vi "粗切.vi"() -> ()   [LabVIEW 2014]
panel:
  out "粗切项目":string
  out "粗切当前状态":string
  out "粗切条码":string
  out "粗切工位生产信息":string[][](table)
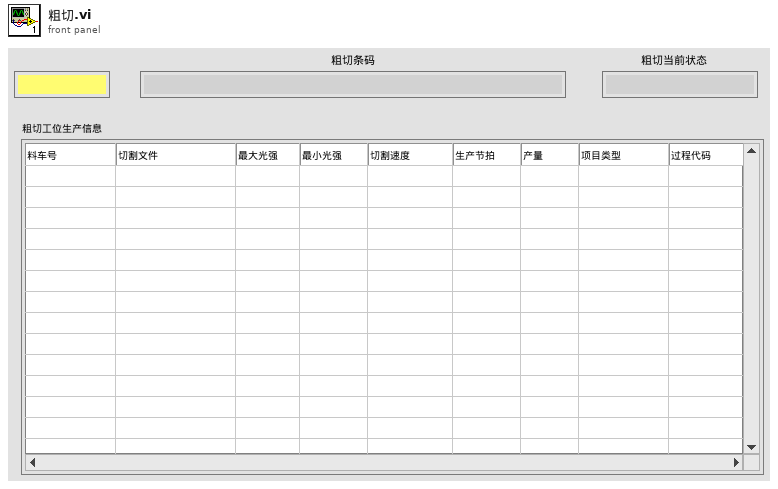
[diagram p1: front panel]
types:
  T1 = cluster{"粗切工位生产信息":refnum<vi>, "粗切条码":refnum<vi>, "粗切当前状态":refnum<vi>, "粗切项目":refnum<vi>}
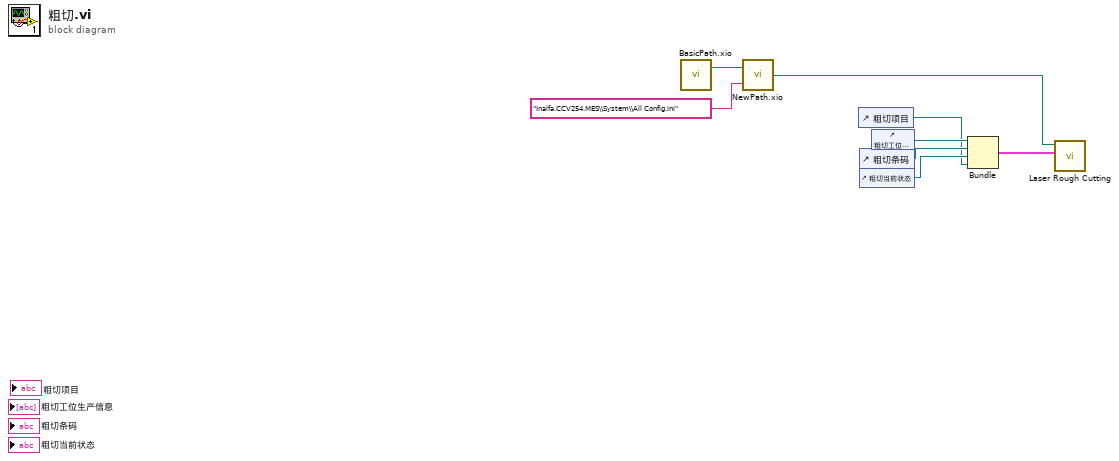
[diagram p0: block diagram]
diagram:
  n1 = call "BasicPath.xio.vi"() -> ("stripped path"=w2:path)  [unwired: 1 in, 1 out]
  n2 = call "NewPath.xio.vi"("Append path"="Inalfa.CCV254.MES\\System\\All Config.ini", "Basic path"=w2) -> ("New path"=w1:path)
  n3 = control-ref of="粗切项目"() -> (w4:refnum<vi>)
  n4 = control-ref of="粗切条码"() -> (w7:refnum<vi>)
  n5 = control-ref of="粗切当前状态"() -> (w6:refnum<vi>)
  n6 = control-ref of="粗切工位生产信息"() -> (w8:refnum<vi>)
  n7 = Bundle("粗切工位生产信息"=w8, "粗切条码"=w7, "粗切当前状态"=w6, "粗切项目"=w4) -> (w5:T1)  [unwired: 1 in]
  n8 = call "Laser Rough Cutting.vi"("configuration file path"=w1, "rough cutting msic"=w5) -> ()  [unwired: 4 in]
